vi "WriteToStringPanel.vi"(10 "String":string, 11 "Ctl Refnum":refnum<vi>) -> ()   [LabVIEW 2017]
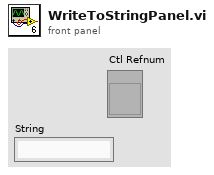
[diagram p1: front panel]
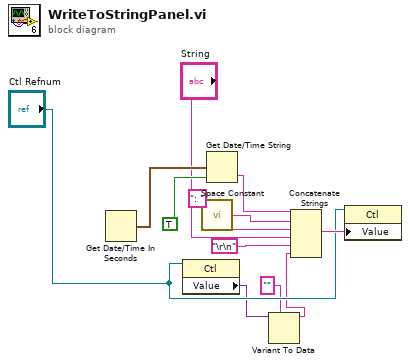
[diagram p0: block diagram]
diagram:
  n1 = Get Date/Time In Seconds() -> (seconds since 1Jan1904=w7:timestamp)
  n2 = property class="Ctl"(reference="Ctl Refnum") -> ("Value"=w3:variant)  [unwired: 1 in, 2 out]
  n3 = call <vilib>:"Space Constant.vi"() -> ("String"=w11:string)
  n4 = Get Date/Time String(seconds (now)=w7, want seconds? (F)=TRUE) -> (time string=w9:string)  [unwired: 1 in, 1 out]
  n5 = Variant To Data(type="", Variant=w3) -> (data=w1:string)  [unwired: 1 in, 1 out]
  n6 = Concatenate Strings(w9, w11, ": ", "String", "\r\n", w1) -> (w10:string)
  n7 = property class="Ctl"(reference="Ctl Refnum", "Value"=w10) -> ()  [unwired: 1 in, 2 out]
